vi "LoadData.vi"(11 "File":path) -> (0 "Rel_T0":timestamp, 1 "I":dbl[](array[numeric]), 2 "V":dbl[](array[numeric]), 3 "T":dbl[](array[numeric]), 4 "Chart":cluster{dbl[], dbl[]}[](array[cluster]), 5 "Tn":timestamp)   [LabVIEW 2025]
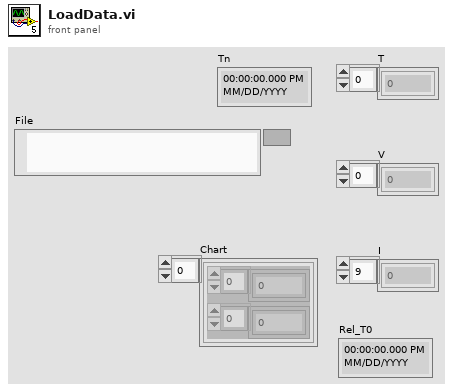
[diagram p1: front panel]
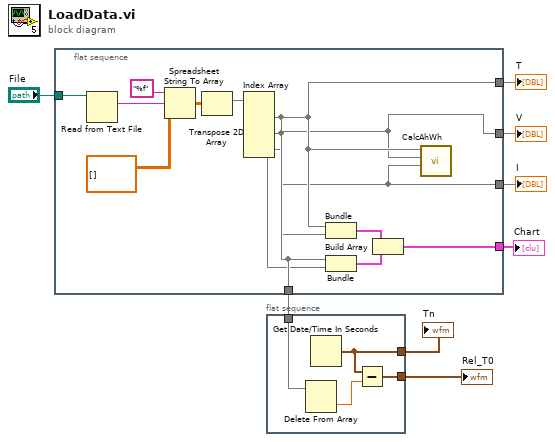
[diagram p0: block diagram]
diagram:
  n1 = flat-sequence {
    tunnel: "File" -> [w20]
    tunnel: [w10] -> w7
    tunnel: [w11] -> w6
    tunnel: [w9] -> w5
    tunnel: [w12] -> w4
    tunnel: [w11] -> w3
    frame #0 {
      n2 = Read from Text File(file (use dialog)=w20) -> (text=w19:string)  [unwired: 3 in, 3 out]
      n3 = Spreadsheet String To Array(format string="%f", spreadsheet string=w19, array type (2D Dbl)=dbl[][] []) -> (array=w16:dbl[][])  [unwired: 1 in]
      n4 = Transpose 2D Array(2D array=w16) -> (transposed array=w15:dbl[][])
      n5 = Index Array(array=w15) -> (element #1=w11:dbl[], element #2=w10:dbl[], element #3=w9:dbl[])  [unwired: 6 in]
      n6 = Bundle(w11, w10) -> (w14:cluster{dbl[], dbl[]})  [unwired: 1 in]
      n7 = Bundle(w11, w9) -> (w13:cluster{dbl[], dbl[]})  [unwired: 1 in]
      n8 = Build Array(w14, w13) -> (w12:cluster{dbl[], dbl[]}[])
      n9 = call "CalcAhWh.vi"("I"=w9, "V"=w10, "T"=w11) -> ()  [unwired: 9 in]
    }
  }
  n10 = flat-sequence {
    tunnel: w3 -> [w24]
    tunnel: [w22] -> w2
    tunnel: [w21] -> w1
    frame #0 {
      n11 = Delete From Array(array=w24) -> (deleted portion=w23:dbl)  [unwired: 2 in, 1 out]
      n12 = Get Date/Time In Seconds() -> (seconds since 1Jan1904=w21:timestamp)
      n13 = Subtract(x=w21, y=w23) -> (x-y=w22:timestamp)
    }
  }
  "Rel_T0" <- w2
  "I" <- w5
  "V" <- w7
  "T" <- w6
  "Chart" <- w4
  "Tn" <- w1
